vi "Configure Waveform Points.vi"(4 "Line End Value (8191)":i32=8191, 5 "Value (8191)":i32=8191, 6 "Line End Index (100)":i32=100, 7 "Index (1)":i32=1, 8 "error in (no error)":errorcluster, 9 "Memory Name (0: Edit Memory)":i32(ring) items=["Edit Memory", "Edit Memory 1", "Edit Memory 2"], 10 "Operation Select (0: Set Point Value)":i32(ring) items=["Set Point Value", "Set Line Value"], 11 "VISA resource name":refnum<visa-resource-name>) -> (0 "error out":errorcluster, 3 "VISA resource name out":refnum<visa-resource-name>)   [LabVIEW 2013, in "Tektronix AFG 3000 Series.lvlib"]
doc: "Sets the data value at specified point index.\n\n<B>Note:</B> \n\nThis VI is only applicable for AFG 3KC series."
uses:
  Tektronix AFG 3000 Series.lvlib
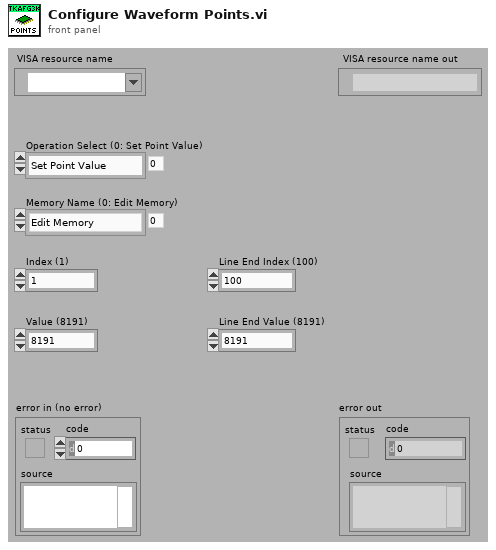
[diagram p1: front panel]
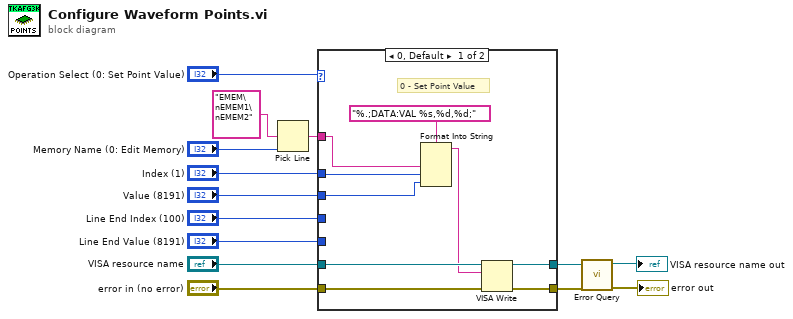
[diagram p0: block diagram]
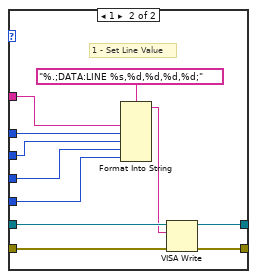
[diagram p2: hidden frame]
diagram:
  n1 = Pick Line(multi-line string="EMEM\nEMEM1\nEMEM2" ("string (\"\")"), line index="Memory Name (0: Edit Memory)") -> (output string=w11:string)  [unwired: 1 in]
  n2 = case shown="0, Default" "Operation Select (0: Set Point Value)" {
    tunnel: w11 -> [w22 w29]
    tunnel: "Index (1)" -> [w21 w28]
    tunnel: "Value (8191)" -> [w20 w27]
    tunnel: "VISA resource name" -> [w19 w34]
    tunnel: "error in (no error)" -> [w18 w33]
    tunnel: [w17 w31] -> w4
    tunnel: [w16 w32] -> w2
    tunnel: "Line End Index (100)" -> [_ w26]
    tunnel: "Line End Value (8191)" -> [_ w25]
    frame 0, Default {
      # "0 - Set Point Value"
      n3 = Format Into String(format string="%.;DATA:VAL %s,%d,%d;", w22, w21, w20) -> (resulting string=w15:string)  [unwired: 2 in, 1 out]
      n4 = VISA Write(VISA resource name=w19, write buffer=w15, error in (no error)=w18) -> (VISA resource name out=w17:refnum<visa-resource-name>, error out=w16:errorcluster)  [unwired: 1 out]
    }
    frame 1 {
      # "1 - Set Line Value"
      n5 = Format Into String(format string="%.;DATA:LINE %s,%d,%d,%d,%d;", w29, w28, w27, w26, w25) -> (resulting string=w24:string)  [unwired: 2 in, 1 out]
      n6 = VISA Write(VISA resource name=w34, write buffer=w24, error in (no error)=w33) -> (VISA resource name out=w31:refnum<visa-resource-name>, error out=w32:errorcluster)  [unwired: 1 out]
    }
  }
  n7 = call "Error Query.vi"("error in (no error)"=w2, "VISA resource name"=w4) -> ("error out"=→"error out":errorcluster, "VISA resource name out"=→"VISA resource name out":refnum<visa-resource-name>)  [unwired: 6 in, 2 out]
